vi "Continuous Audio Output Example.vi"() -> ()   [LabVIEW 2020]
doc: "Simple example of continuous audio output of a file decoded with G-Audio and passed to LabVIEW's sound device VIs."
uses:
  <vilib>/sound2/lvsound2.llb/Sampling Mode.ctl
  <vilib>/sound2/lvsound2.llb/Sound Data Format.ctl
  8289e2ef-86ba-4438-8a42-485f00fd8c95.vi
  27920591-b795-4816-8ad5-c0c2393af623.vi
  Private/Get Basic Audio File Info.vi
  Private/Result To Error.vi
  8289e2ef-86ba-4438-8a42-485f00fd8c95.vi/779dfdfd-1b42-4cf4-8001-66d3dd167625.vi
  8289e2ef-86ba-4438-8a42-485f00fd8c95.vi/55d550d4-9624-414e-aebd-6e02b5081896.vi
  8289e2ef-86ba-4438-8a42-485f00fd8c95.vi/779dfdfd-1b42-4cf4-8001-66d3dd167625.vi/a9d2058a-38f9-4c88-a1a9-9bf864ebbde5.vi
  8289e2ef-86ba-4438-8a42-485f00fd8c95.vi/55d550d4-9624-414e-aebd-6e02b5081896.vi/4b7b629c-2e91-4160-9820-a26af8f6e677.vi
  8289e2ef-86ba-4438-8a42-485f00fd8c95.vi/55d550d4-9624-414e-aebd-6e02b5081896.vi/e7c4a249-ce38-42b4-8985-5fdb76b4ebfc.vi
  <vilib>/Utility/Data Type/Get Numeric Information.vi
  <vilib>/Utility/error.llb/Error Cluster From Error Code.vi
  <vilib>/sound2/lvsound2.llb/Sound Output Write (I16).vi
  G-Audio.lvlib
panel:
  out "Now Playing:":string
  out "Duration":string
  out "Sample Length":u64
  out "Audio Info":T1
  out "error out":errorcluster
  in  "Stop":bool
  out "Waveform":waveform(i16)[](graph)
  # "Instructions:\n1. Run the VI.\n2. Select an audio file to play.\n3. The VI will stop when the file has finished playing, or when the Stop button is pressed."
  # "G"
  # "-Audio"
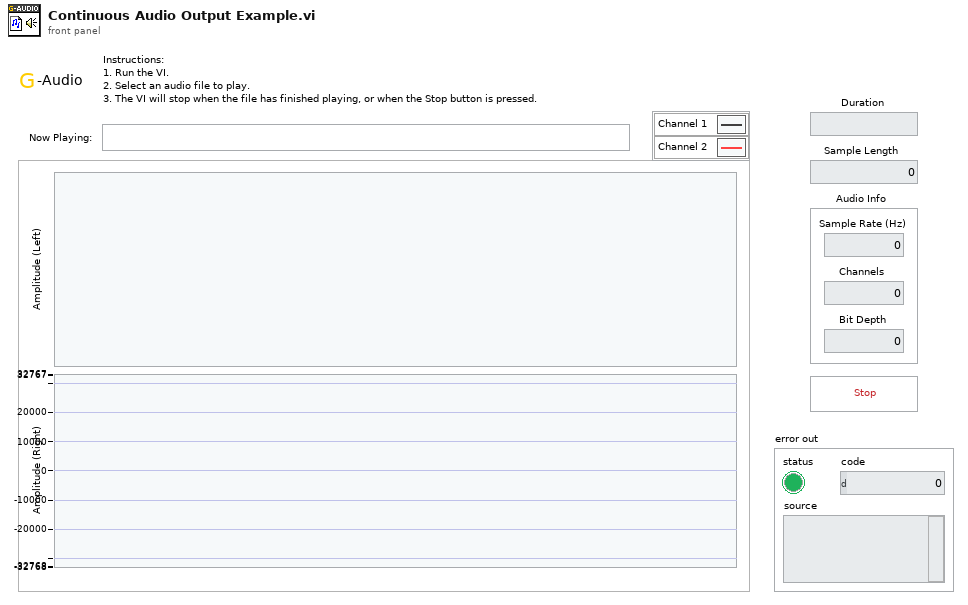
[diagram p1: front panel]
types:
  T1 = cluster{"Sample Rate (Hz)":u32, "Channels":u32, "Bit Depth":u32}
  T2 = typedef "Sound Data Format.ctl" = cluster{"sample rate (S/s)":dbl, "number of channels":i32, "bits per sample":i32}
  T3 = typedef "Sampling Mode.ctl" = i32
  T4 = typedef "G-Audio.lvlib/Audio File Info.ctl" = cluster{"Sample Rate (Hz)":u32, "Channels":u32, "Bit Depth":u32}
  T5 = typedef "Sound Output Task ID.ctl" = u32
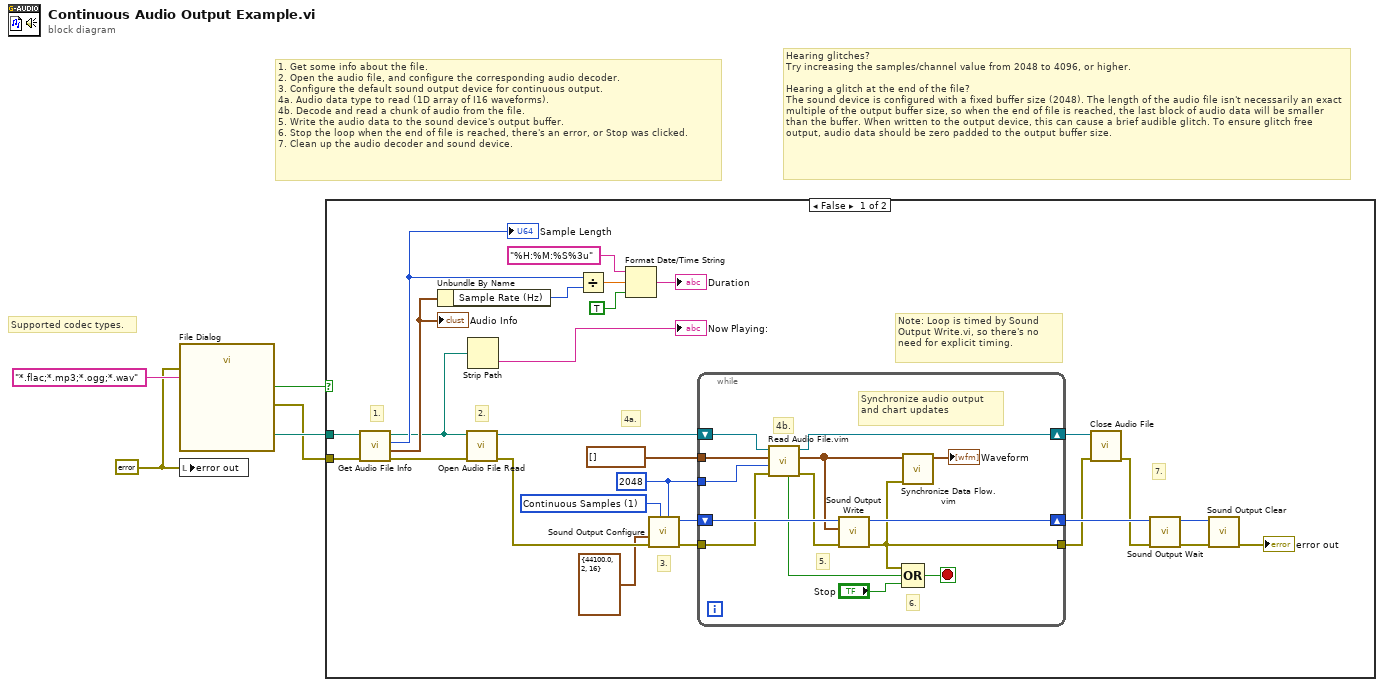
[diagram p0: block diagram]
diagram:
  w1 = errorcluster {"status"=FALSE, "code"=0, "source"=""} ("error out")
  # "Hearing glitches?\nTry increasing the samples/channel value from 2048 to 4096, or higher.\n\nHearing a glitch at the end of the file?\nThe sound device is configured with a fixed buffer size (2048). The length of the audio file isn't necessarily an exact multiple of the output buffer size, so when the end of file is reached, the last block of audio data will be smaller than the buffer. When written to the output device, this can cause a brief audible glitch. To ensure glitch free output, audio data should be zero padded to the output buffer size."
  # "1. Get some info about the file.\n2. Open the audio file, and configure the corresponding audio decoder.\n3. Configure the default sound output device for continuous output.\n4a. Audio data type to read (1D array of I16 waveforms).\n4b. Decode and read a chunk of audio from the file.\n5. Write the audio data to the sound device's output buffer.\n6. Stop the loop when the end of file is reached, there's an error, or Stop was clicked.\n7. Clean up the audio decoder and sound device."
  # "Supported codec types."
  n1 = call "File Dialog"("error in"=w1, "pattern (all files)"="*.flac;*.mp3;*.ogg;*.wav") -> ("selected path"=w4:path, "cancelled"=w3:bool, "error out"=w2:errorcluster)  [unwired: 10 in, 1 out]
  n2 = local write "error out"(w1) -> ()
  n3 = case shown="False" w3 {
    tunnel: w4 -> [w18 _]
    tunnel: w2 -> [w31 _]
    frame False {
      w20 = u64 2048 ("number of samples/ch")
      w32 = T3 1 items=["Finite Samples", "Continuous Samples"] ("sample mode")
      # "Note: Loop is timed by Sound Output Write.vi, so there's no need for explicit timing."
      # "4a."
      # "7."
      # "3."
      # "2."
      # "1."
      n4 = call "Get Audio File Info.vi"("error in (no error)"=w31, "Path In"=w18) -> ("error out"=w30:errorcluster, "Audio File Info"=w12:T4, "Sample Length"=w13:u64, "Path Out"=w7:path)  [unwired: 6 in]
      "Audio Info" <- w12
      "Sample Length" <- w13
      n5 = Unbundle By Name(w12) -> ("Sample Rate (Hz)"=w11:u32)
      n6 = call "Open Audio File Read.vi"("error in (no error)"=w30, "Path"=w7) -> ("error out"=w26:errorcluster, "Audio File Refnum"=w17:refnum<file>)  [unwired: 8 in]
      n7 = Strip Path(path=w7) -> (name=→"Now Playing:":string)  [unwired: 1 out]
      n8 = Divide(x=w13, y=w11) -> (x/y=w10:dbl)
      n9 = Format Date/Time String(time format string (%c)="%H:%M:%S%3u", seconds (now)=w10, UTC format=TRUE) -> (date/time string=→"Duration":string)
      n10 = call <vilib>:"Sound Output Configure.vi"("number of samples/ch"=w20, "sample mode"=w32, "error in (no error)"=w26, "sound format"=T2 {"sample rate (S/s)"=44100.0, "number of channels"=2, "bits per sample"=16}) -> ("error out"=w21:errorcluster, "task ID"=w22:T5)  [unwired: 6 in]
      n11 = while {
        shift-right: [w44] -> w29
        shift-left: w17 -> [w46]
        shift-right: [w43] -> w28
        shift-left: w22 -> [w45]
        tunnel: w21 -> [w42]
        tunnel: [w36] -> w25
        tunnel: w20 -> [w35]
        tunnel: waveform(i16)[] [] -> [w33]
        stop <- w39 stop-if-true
        # "Synchronize audio output and chart updates"
        # "6."
        # "5."
        # "4b."
        n12 = call "Read Audio File.vim"("error in (no error)"=w42, "Samples To Read"=w35, "Data Format"=w33, "Audio File Refnum In"=w46) -> ("error out"=w41:errorcluster, "Audio Data"=w34:waveform(i16)[], "Audio File Refnum Out"=w44:refnum<file>, "End of File?"=w40:bool)  [unwired: 3 in, 1 out]
        n13 = call-poly <vilib>:"Sound Output Write.vi"("error in (no error)"=w41, "data"=w34, "task ID"=w45) -> ("error out"=w36:errorcluster, "task ID out"=w43:T5)  [unwired: 7 in]
        n14 = Compound Arithmetic op=OR(w36, w40, "Stop") -> (w39:bool)
        n15 = call "Synchronize Data Flow.vim"("input 4"=w36, "input 1"=w34) -> ("output 1"=→"Waveform":waveform(i16)[])  [unwired: 2 in, 3 out]
      }
      n16 = call "Close Audio File.vi"("error in (no error)"=w25, "Audio File Refnum In"=w29) -> ("error out"=w24:errorcluster)  [unwired: 9 in]
      n17 = call <vilib>:"Sound Output Wait.vi"("error in (no error)"=w24, "task ID"=w28) -> ("error out"=w23:errorcluster, "task ID out"=w27:T5)  [unwired: 8 in]
      n18 = call <vilib>:"Sound Output Clear.vi"("error in (no error)"=w23, "task ID"=w27) -> ("error out"=→"error out":errorcluster)  [unwired: 9 in]
    }
    frame True {
    }
  }
